vi "Insert Watermark.vi"(0 "OverContent":refnum<k24>, 9 "Watermark Cluster":T1={"Show? (F)"=TRUE, "Type"=enum."Image", "Opacity (%)"=10.0, "Rotate(°)"=0.0, "Position"={"Position"=enum."Center (text section)", "X"=0.0, "Y"=0.0}, "Image path"=path "", "Scaled(%)"=100.0, "Image refnum"=refnum, "Text"="CONFIDENTIAL", "Font"={"Name"="", "Size"=-1.0, "Color"=0}, "Font refnum"=refnum, "Alignment"=enum."Center", "Automatic"=FALSE}, 11 "error in (no error)":errorcluster) -> (4 "OverContent duplicate":refnum<k24>, 15 "error out":errorcluster)   [LabVIEW 2012]
doc: "Version 1.0\nDeveloped by Jean-Marc Simard\nCopyright © 2010, Exaprom Inc.\nAll rights reserved.\nLicense: BSD\n\nWith iTextSharp 4.1.6 (http://itextsharp.sourceforge.net)\nunder Mozilla Public License Version 1.1\n(http://www.mozilla.org/MPL/MPL-1.1.html)"
uses:
  C:/Users/MaxCorp/Documents/TopPerm - Base/DLL/itextsharp.dll
  DLL/itextsharp.dll
  Controls/Watermark cluster2.ctl
  Controls/Watermark Position.ctl
  Controls/Font size.ctl
  Controls/Font color.ctl
  Controls/Header footer horiz alignment.ctl
  Controls/CB SetColor.ctl
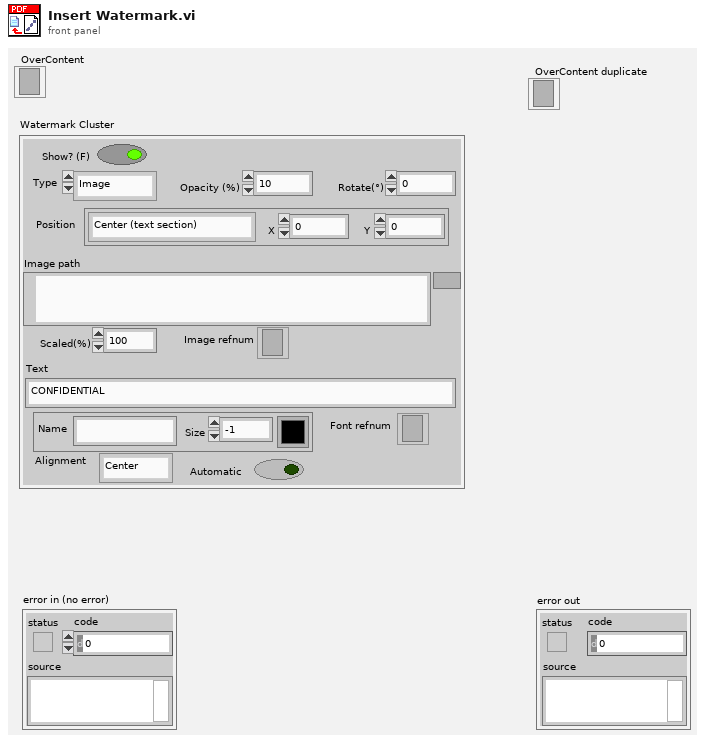
[diagram p1: front panel]
types:
  T1 = typedef "Watermark cluster2.ctl" = cluster{"Show? (F)":bool, "Type":enum16{"Image", "Text"}, "Opacity (%)":sgl, "Rotate(°)":sgl, "Position":cluster{"Position":T2, "X":sgl, "Y":sgl}, "Image path":path, "Scaled(%)":sgl, "Image refnum":refnum<k24>, "Text":string, "Font":cluster{"Name":string, "Size":T3, "Color":T4}, "Font refnum":refnum<k24>, "Alignment":T5, "Automatic":bool}
  T2 = typedef "Watermark Position.ctl" = enum16{"Absolute", "Center (page)", "Center (text section)"}
  T3 = typedef "Font size.ctl" = sgl
  T4 = typedef "Font color.ctl" = u32
  T5 = typedef "Header footer horiz alignment.ctl" = enum16{"Left", "Center", "Right"}
  T6 = typedef "CB SetColor.ctl" = enum16{"Fill", "Stroke"}
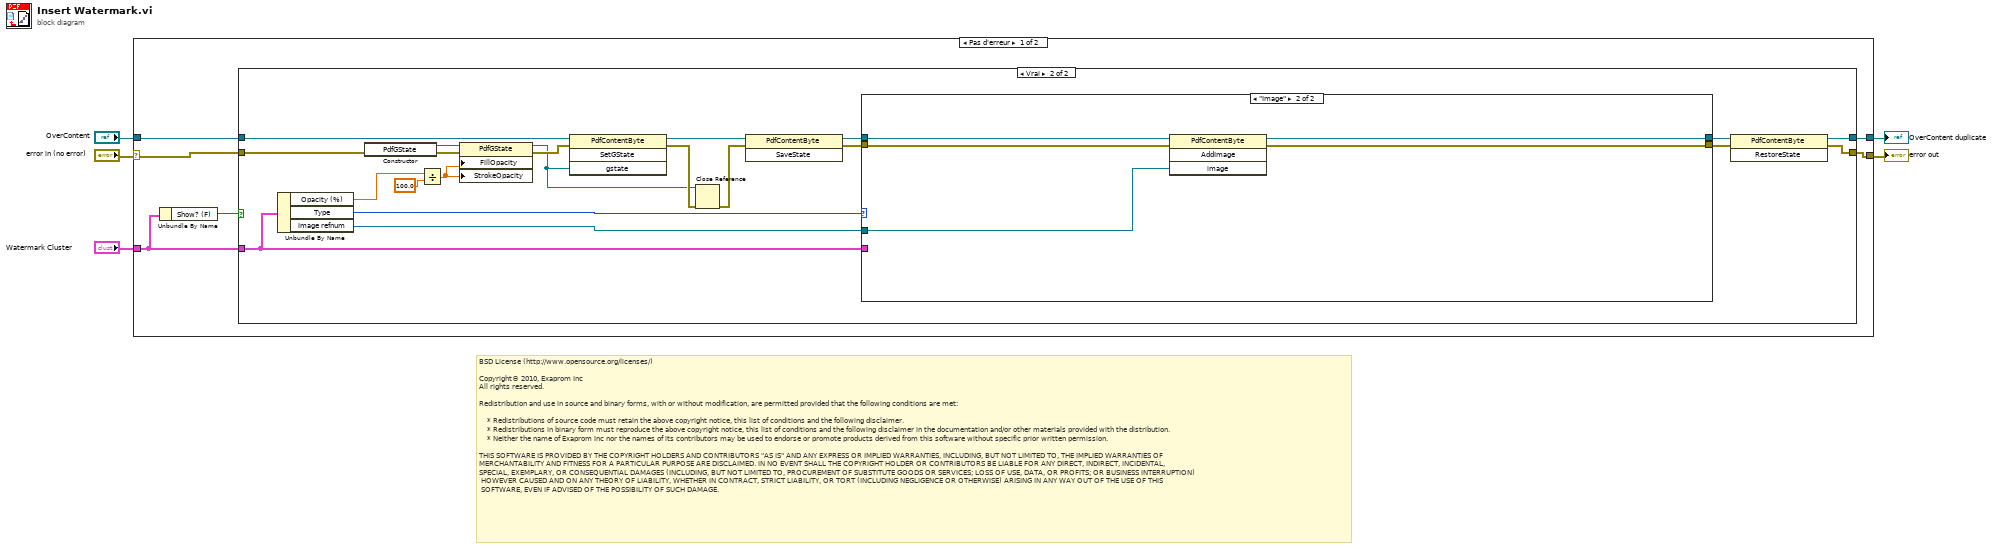
[diagram p0: block diagram]
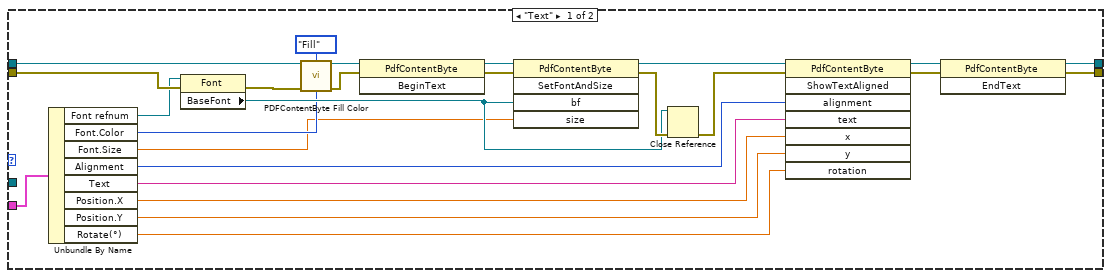
[diagram p3: hidden frame]
diagram:
  # "BSD License (http://www.opensource.org/licenses/)\n\nCopyright© 2010, Exaprom Inc\nAll rights reserved.\n\nRedistribution and use in source and binary forms, with or without modification, are permitted provided that the following conditions are met:\n\n    * Redistributions of source code must retain the above copyright notice, this list of conditions and the following disclaimer.\n    * Redistributions in binary form must reproduce the above copyright notice, this list of conditions and the following disclaimer in the documentation and/or other materials provided with the distribution.\n    * Neither the name of Exaprom Inc nor the names of its contributors may be used to endorse or promote products derived from this software without specific prior written permission.\n\nTHIS SOFTWARE IS PROVIDED BY THE COPYRIGHT HOLDERS AND CONTRIBUTORS \"AS IS\" AND ANY EXPRESS OR IMPLIED WARRANTIES, INCLUDING, BUT NOT LIMITED TO, THE IMPLIED WARRANTIES OF \nMERCHANTABILITY AND FITNESS FOR A PARTICULAR PURPOSE ARE DISCLAIMED. IN NO EVENT SHALL THE COPYRIGHT HOLDER OR CONTRIBUTORS BE LIABLE FOR ANY DIRECT, INDIRECT, INCIDENTAL,\nSPECIAL, EXEMPLARY, OR CONSEQUENTIAL DAMAGES (INCLUDING, BUT NOT LIMITED TO, PROCUREMENT OF SUBSTITUTE GOODS OR SERVICES; LOSS OF USE, DATA, OR PROFITS; OR BUSINESS INTERRUPTION)\n HOWEVER CAUSED AND ON ANY THEORY OF LIABILITY, WHETHER IN CONTRACT, STRICT LIABILITY, OR TORT (INCLUDING NEGLIGENCE OR OTHERWISE) ARISING IN ANY WAY OUT OF THE USE OF THIS\n SOFTWARE, EVEN IF ADVISED OF THE POSSIBILITY OF SUCH DAMAGE."
  n1 = case shown="Pas d'erreur" "error in (no error)" {
    selector: "error in (no error)" -> [w10 w66]
    tunnel: [w8 w66] -> w4
    tunnel: "OverContent" -> [w11 w65]
    tunnel: [w9 w65] -> w2
    tunnel: "Watermark Cluster" -> [w7 _]
    frame No Error {
      n2 = Unbundle By Name(w7) -> ("Show? (F)"=w6:bool)
      n3 = case shown="Vrai" w6 {
        tunnel: w11 -> [w13 w20]
        tunnel: w10 -> [w12 w34]
        tunnel: [w13 w33] -> w9
        tunnel: [w12 w32] -> w8
        tunnel: w7 -> [_ w21]
        frame False {
        }
        frame True {
          n4 = Unbundle By Name(w21) -> ("Opacity (%)"=w22:sgl, "Type"=w31:enum16{"Image", "Text"}, "Image refnum"=w14:refnum<k24>)
          n5 = constructor class="PdfGState"(error in=w34) -> (reference out=w17:refnum<k24>, error out=w18:errorcluster)  [unwired: 2 in, 1 out]
          n6 = Divide(x=w22, y=sgl 100.0) -> (x/y=w15:sgl)
          n7 = property class="PdfGState"(reference=w17, error in=w18, "FillOpacity"=w15, "StrokeOpacity"=w15) -> (reference out=w19:refnum<k24>, error out=w27:errorcluster)
          n8 = invoke class="PdfContentByte" method="SetGState"(reference=w20, error in=w27, "gstate"=w19) -> (reference out=w26:refnum<k24>, error out=w28:errorcluster)  [unwired: 1 in, 2 out]
          n9 = Close Reference(reference=w19, error in (no error)=w28) -> (error out=w24:errorcluster)
          n10 = invoke class="PdfContentByte" method="SaveState"(reference=w26, error in=w24) -> (reference out=w25:refnum<k24>, error out=w23:errorcluster)  [unwired: 1 in, 1 out]
          n11 = case shown="\"Image\"" w31 {
            tunnel: w25 -> [w44 w63]
            tunnel: [w49 w64] -> w30
            tunnel: [w48 w61] -> w29
            tunnel: w23 -> [w40 w62]
            tunnel: w21 -> [w50 _]
            tunnel: w14 -> [_ w60]
            frame "Text" {
              n12 = Unbundle By Name(w50) -> ("Font refnum"=w39:refnum<k24>, "Font.Color"=w36:T4, "Font.Size"=w35:T3, "Alignment"=w52:T5, "Text"=w42:string, "Position.X"=w56:sgl, "Position.Y"=w55:sgl, "Rotate(°)"=w37:sgl)
              n13 = property class="Font"(reference=w39, error in=w40) -> (error out=w38:errorcluster, "BaseFont"=w47:refnum<k24>)  [unwired: 1 out]
              n14 = call "PDFContentByte Fill Color.vi"("PDFContentByte"=w44, "CB SetColor"=CB_SetColor."Fill", "error in (no error)"=w38, "Color Box"=w36) -> ("PDFContentByte duplicate"=w46:refnum<k24>, "error out"=w45:errorcluster)  [unwired: 10 out]
              n15 = invoke class="PdfContentByte" method="BeginText"(reference=w46, error in=w45) -> (reference out=w58:refnum<k24>, error out=w59:errorcluster)  [unwired: 1 in, 1 out]
              n16 = invoke class="PdfContentByte" method="SetFontAndSize"(reference=w58, error in=w59, "bf"=w47, "size"=w35) -> (reference out=w41:refnum<k24>, error out=w54:errorcluster)  [unwired: 1 in, 3 out]
              n17 = Close Reference(reference=w47, error in (no error)=w54) -> (error out=w53:errorcluster)
              n18 = invoke class="PdfContentByte" method="ShowTextAligned"(reference=w41, error in=w53, "alignment"=w52, "text"=w42, "x"=w56, "y"=w55, "rotation"=w37) -> (reference out=w51:refnum<k24>, error out=w57:errorcluster)  [unwired: 1 in, 6 out]
              n19 = invoke class="PdfContentByte" method="EndText"(reference=w51, error in=w57) -> (reference out=w49:refnum<k24>, error out=w48:errorcluster)  [unwired: 1 in, 1 out]
            }
            frame "Image" {
              n20 = invoke class="PdfContentByte" method="AddImage"(reference=w63, error in=w62, "image"=w60) -> (reference out=w64:refnum<k24>, error out=w61:errorcluster)  [unwired: 1 in, 2 out]
            }
          }
          n21 = invoke class="PdfContentByte" method="RestoreState"(reference=w30, error in=w29) -> (reference out=w33:refnum<k24>, error out=w32:errorcluster)  [unwired: 1 in, 1 out]
        }
      }
    }
    frame Error {
    }
  }
  "error out" <- w4
  "OverContent duplicate" <- w2
